vi "Set Sessions AWG.vi"(0 "Semiconductor Module Context":T1, 3 "error in (no error)":errorcluster) -> (7 "Semiconductor Module Context Out":T1, 8 "Instrument Array":refnum<k15>[](array[refnum]), 10 "error out":errorcluster)   [LabVIEW 2013]
uses:
  <vilib>/NI_TestStand_SemiconductorModule/NI_TestStand_Semiconductor_Module.lvlibp/PinMap/General/SemiconductorModuleContext.ctl
  <vilib>/NI_TestStand_SemiconductorModule/NI_TestStand_Semiconductor_Module.lvlibp
panel:
  out "Channel Lists":string[](array[string])
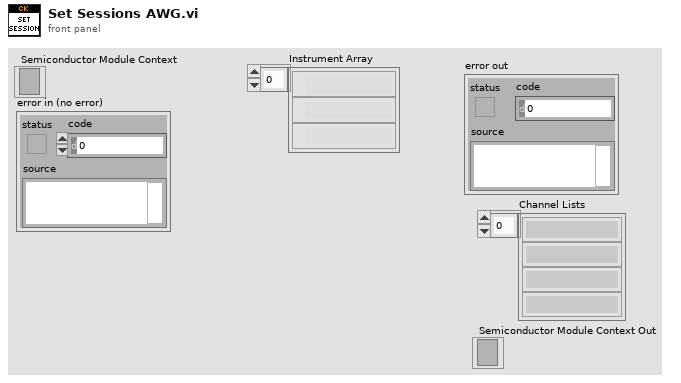
[diagram p1: front panel]
types:
  T1 = typedef "NI_TestStand_Semiconductor_Module.lvlibp/SemiconductorModuleContext.ctl" = refnum<k7>
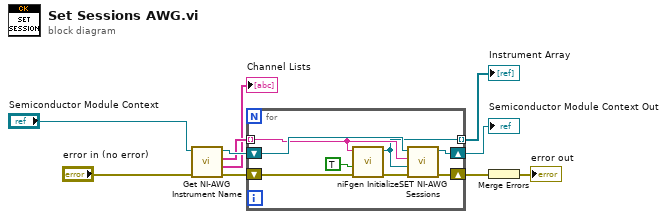
[diagram p0: block diagram]
diagram:
  n1 = call "Get NI-AWG Instrument Name.vi"("Semiconductor Module Context"="Semiconductor Module Context", "error in (no error)"="error in (no error)") -> ("Semiconductor Module Context Out"=w8:T1, "Instrument Names"=w6:string[], "Channel Lists"=→"Channel Lists":string[], "error out"=w7:errorcluster)  [unwired: 5 in]
  n2 = for {
    shift-right: [w17] -> w9
    shift-left: w7 -> [w18]
    tunnel: w6 -> [w14] mode=indexing
    shift-right: [w16] -> w1
    shift-left: w8 -> [w15]
    tunnel: [w12] -> w4 mode=indexing
    n3 = call <instrlib>:"niFgen Initialize.vi"("error in (no error)"=w18, "Reset Device (default: True)"=TRUE, "Resource Name"=w14) -> ("error out"=w13:errorcluster, "Instrument Handle Out"=w12:refnum<k15>)  [unwired: 7 in]
    n4 = call "SET NI-AWG Sessions.vi"("error in (no error)"=w13, "Instrument Handle In"=w12, "Instrument Name"=w14, "Semiconductor Module Context"=w15) -> ("error out"=w17:errorcluster, "Semiconductor Module Context Out"=w16:T1)  [unwired: 6 in]
  }
  "Instrument Array" <- w4
  "Semiconductor Module Context Out" <- w1
  n5 = Merge Errors(w9) -> (→"error out":errorcluster)
